vi "AIScale.vi"(0 "B":i16[](array[numeric])=[0, 0, 0, 0, 0, 0, 0, 0, 0, 0, 0, 0, 0, 0, 0, 0], 5 "M":sgl[](array[numeric])=[0.0, 0.0, 0.0, 0.0, 0.0, 0.0, 0.0, 0.0, 0.0, 0.0, 0.0, 0.0, 0.0, 0.0, 0.0, 0.0], 7 "UnscaledAI":i16[](array[numeric])=[0, 0, 0, 0, 0, 0, 0, 0, 0, 0, 0, 0, 0, 0, 0, 0], 11 "index":u8) -> (4 "ScaledAI":sgl[](array[numeric]))   [LabVIEW 2017, in "ScaleAndLimit.lvlib"]
uses:
  ScaleAndLimit.lvlib
  <vilib>/rvi/IPIntegrationNode/IPINode_Typedef/niFpgaIPINodeSupportedFamilies.ctl
  <userlib>/_NI FLP Library/FPGA/insideSCTL/FlpLib Multiply SCTL Latency 0.vi
  <vilib>/rvi/IPIntegrationNode/IPINode_Utilities/niFpgaIPINodeSimCore.vi
  <vilib>/rvi/XilinxIP/XIPIN_XNode/niFpgaXIPIN.xnode
  AIScale/I16ToSGL_convert/xsim.dir/I16ToSGL_convert_BAEB0EFF4B15497ABBB37471944D9EC5/xsimk_BAEB0EFF4B15497ABBB37471944D9EC5.dll
  <vilib>/rvi/IPIntegrationNode/IPINode_Xnode/niFpgaIPINode.xnode
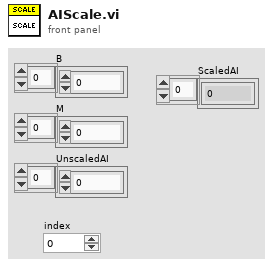
[diagram p1: front panel]
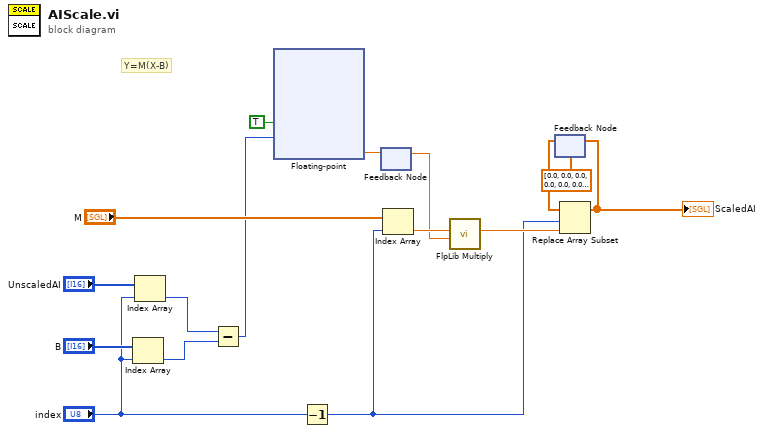
[diagram p0: block diagram]
diagram:
  # "Y=M(X-B)"
  n1 = Index Array(array="B", index="index") -> (element=w12:i16)
  n2 = Index Array(array="UnscaledAI", index="index") -> (element=w13:i16)
  n3 = Subtract(x=w13, y=w12) -> (x-y=w5:i16)
  n4 = xnode ("Floating-point")("s_axis_a_tvalid"=TRUE, "s_axis_a_tdata"=w5) -> ("m_axis_result_tdata"=w4:sgl)  [unwired: 1 out]
  n5 = Decrement(x="index") -> (x-1=w1:u8)
  n6 = feedback-in #1(w4) -> ()
  n7 = feedback #1() -> (w3:sgl)  [unwired: 1 in]
  n8 = Index Array(array="M", index=w1) -> (element=w11:sgl)
  n9 = call-poly <userlib>:"FlpLib Multiply.vi"("y"=w3, "x"=w11) -> ("x*y"=w8:sgl)  [unwired: 5 in]
  n10 = feedback #2(sgl[] [0.0, 0.0, 0.0, 0.0, 0.0, 0.0, 0.0, 0.0, 0.0, 0.0, 0.0, 0.0, 0.0, 0.0, 0.0, 0.0] ("ScaledAI 2")) -> (w9:sgl[])
  n11 = Replace Array Subset(array=w9, new element=w8, index=w1) -> (w7:sgl[])
  "ScaledAI" <- w7
  n12 = feedback-in #2(w7) -> ()
